vi "Visa_Write read_UI SETPIN.vi"(0 "Simulado in":refnum<class "Simulado.lvclass">, 1 "VISA Refnum in":refnum<visa-resource-name>, 3 "Command to Send":string, 5 "error in (no error)":errorcluster) -> (14 "Simulado out":refnum<class "Simulado.lvclass">, 15 "VISA Refnum out":refnum<visa-resource-name>, 16 "Puerto":string, 17 "Valor Pin":string, 18 "Pin":bool, 19 "error out":errorcluster)   [LabVIEW 2020, in "Simulado.lvclass"]
uses:
  Simulado.lvclass
  Abstract/Serial Device/Combo Box Devices.ctl
  Abstract/Serial Device/Combo Box Comandos.ctl
  UI Actor/UI Actor.lvclass
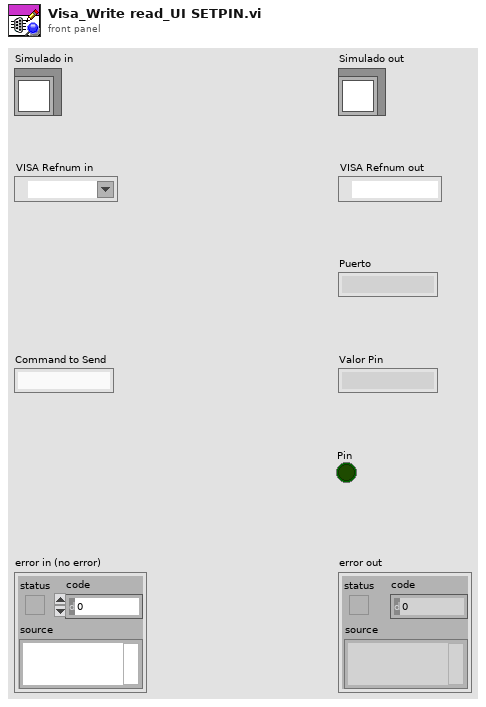
[diagram p1: front panel]
types:
  T1 = typedef "Combo Box Comandos.ctl" = string
  T2 = typedef "Combo Box Devices.ctl" = string
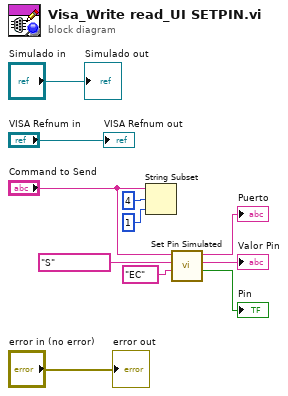
[diagram p0: block diagram]
diagram:
  n1 = String Subset(string="Command to Send", offset (0)=4, length (rest)=1 ("offset (0)")) -> ()  [unwired: 1 out]
  n2 = call "Set Pin Simulated.vi"("Command"=T1 "EC", "Serial Devide Brand"=T2 "S", "Command to Send"="Command to Send") -> ("Pin"=→"Pin":bool, "Valor Pin"=→"Valor Pin":string, "Puerto"=→"Puerto":string)  [unwired: 6 in]
  "error out" <- "error in (no error)"
  "Simulado out" <- "Simulado in"
  "VISA Refnum out" <- "VISA Refnum in"
